vi "Init Hardware.vi"(8 "error in (no error)":errorcluster, 11 "Red Pitaya Digitizer in":refnum<class "Red Pitaya Digitizer.lvclass">) -> (0 "error out":errorcluster, 3 "Red Pitaya Digitizer out":refnum<class "Red Pitaya Digitizer.lvclass">)   [LabVIEW 2018, in "Red Pitaya Digitizer.lvclass"]
uses:
  Red Pitaya Digitizer.lvclass
  C:/github/NHMFL_Core/Libraries/Instruments/Pulse Driver/Pulse Driver.lvclass
  Red Pitaya Digitizer.lvclass/Red Pitaya Digitizer.ctl
  Instruments/Pulse Driver/Pulse Driver.lvclass/Pulse Driver.ctl
  RP Core/RP Instrument/RP Instrument.lvclass/RP Instrument.ctl
  RP Command.ctl
  Read Logic tag.vi
  Read RP Instrument.vi
  Instruments/Pulse Driver/Read Samples per channel.vi
  Instruments/Pulse Driver/Read Pretrigger samples.vi
  Read Tigger level.vi
  RP Core/RP Instrument/Write Decimation.vi
  RP Core/RP Instrument/Write Post-trigger samples.vi
  RP Core/RP Instrument/Write Samples per trigger increment .vi
  Write RP Instrument.vi
  Instruments/Pulse Driver/Write dt.vi
  Instruments/Pulse Driver/Write t0.vi
  Write Signal bits.vi
  Read Server address.vi
  RP Core/RP Instrument/RP Instrument.lvclass
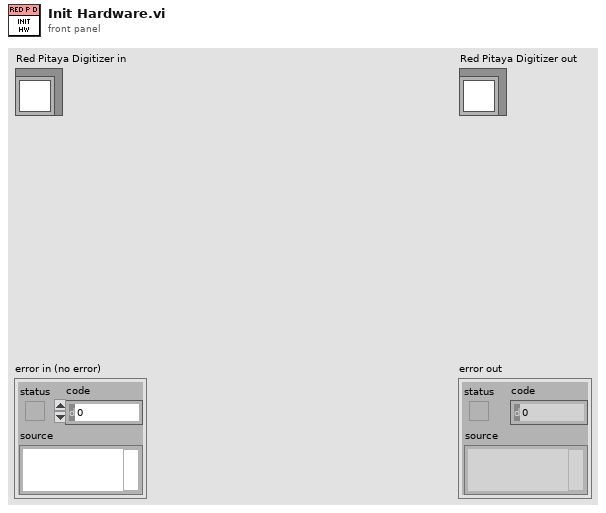
[diagram p1: front panel]
types:
  T1 = typedef "RP Command.ctl" = enum16{"Reset", "Read IDN", "Stop server", "Get status", "Get temperature", "Connect client", "Arm", "Software trigger", "Get whole buffer", "Get chunk", "System call", "Get config", "Set config", "Recieve data", "Recieve Calibartion", "Transmit data"}
  T2 = typedef "Pusle Driver Configuration.ctl" = cluster{"Pre-trigger duration":dbl, "Post-trigger duration":dbl, "Rate":dbl, "Ranges":dbl[], "Re-name channels":string[], "Active channels":string, "External clock":bool}
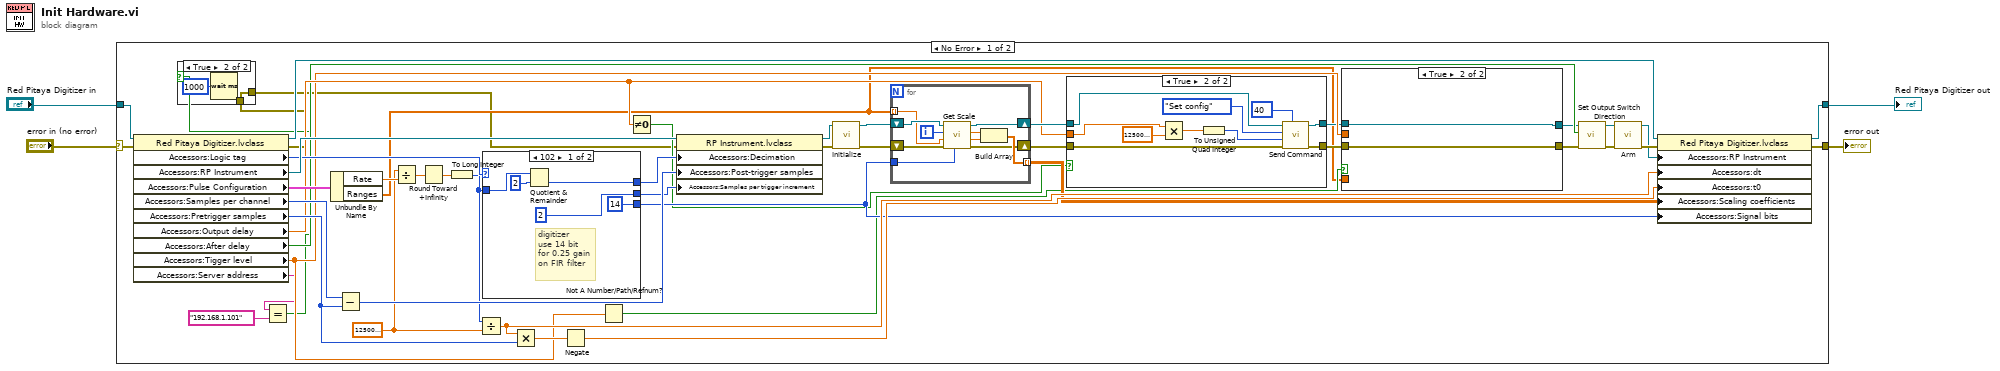
[diagram p0: block diagram]
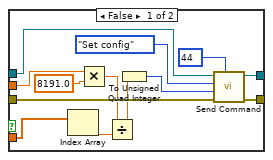
[diagram p3: hidden frame]
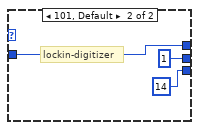
[diagram p5: hidden frame]
diagram:
  n1 = case shown="No Error" "error in (no error)" {
    selector: "error in (no error)" -> [w32 w101]
    tunnel: "Red Pitaya Digitizer in" -> [w52 w102]
    tunnel: [w40 w101] -> w2
    tunnel: [w39 w102] -> w1
    frame No Error {
      w38 = 125000000.0 ("y")
      n2 = property class="Red Pitaya Digitizer.lvclass"(reference=w52, error in=w32) -> (reference out=w42:refnum<class "Red Pitaya Digitizer.lvclass">, error out=w6:errorcluster, "Accessors:Logic tag"=w28:u16, "Accessors:RP Instrument"=w31:refnum<class "RP Instrument.lvclass">, "Accessors:Pulse Configuration"=w51:T2, "Accessors:Samples per channel"=w46:i32, "Accessors:Pretrigger samples"=w36:u32, "Accessors:Output delay"=w20:dbl, "Accessors:After delay"=w17:bool, "Accessors:Tigger level"=w12:dbl, "Accessors:Server address"=w9:string)
      n3 = Equal?(x=w9, y="192.168.1.101") -> (x = y?=w7:bool)
      n4 = case shown="True" w7 {
        tunnel: w6 -> [w53 w54]
        tunnel: [w53 w54] -> w5
        frame False {
        }
        frame True {
          n5 = Wait (ms)(milliseconds to wait=u32 1000) -> ()  [unwired: 1 out]
        }
      }
      n6 = Unbundle By Name(w51) -> ("Rate"=w50:dbl, "Ranges"=w10:dbl[])
      n7 = Subtract(x=w46, y=w36) -> (x-y=w45:u32)
      n8 = Divide(x=w38, y=w50) -> (x/y=w49:dbl)
      n9 = Round Toward +Infinity(x=w49) -> (ceil(x): smallest int >= x=w48:dbl)
      n10 = To Long Integer(number=w48) -> (32bit integer=w27:i32)
      n11 = Divide(x=w27, y=w38) -> (x/y=w37:dbl)
      n12 = case shown="102" w28 {
        tunnel: [14 ("Signal bits") 14 ("Signal bits")] -> w29
        tunnel: [2 ("Samples per trigger increment") 1 ("Samples per trigger increment")] -> w30
        tunnel: w27 -> [w85 w88]
        tunnel: [w83 w88] -> w26
        frame 102 {
          # "digitizer\nuse 14 bit \nfor 0.25 gain\non FIR filter"
          n13 = Quotient & Remainder(x=w85, y=2) -> (floor(x/y)=w83:i32)  [unwired: 1 out]
        }
        frame 101, Default {
          # "lockin-digitizer"
        }
      }
      n14 = Multiply(x=w37, y=w36) -> (x*y=w35:dbl)
      n15 = Negate(x=w35) -> (-x=w34:dbl)
      n16 = Not A Number/Path/Refnum?(number/path/refnum=w12) -> (NaN/Path/Refnum?=w13:bool)
      n17 = Not Equal To 0?(x=w20) -> (x != 0?=w23:bool)
      n18 = property class="RP Instrument.lvclass"(reference=w31, error in=w5, "Accessors:Decimation"=w26, "Accessors:Post-trigger samples"=w45, "Accessors:Samples per trigger increment "=w30) -> (reference out=w47:refnum<class "RP Instrument.lvclass">, error out=w44:errorcluster)
      n19 = call-dynamic "Initialize.vi"("error in (no error)"=w44, "RP Instrument in"=w47) -> ("error out"=w24:errorcluster, "RP Instrument out"=w25:refnum<class "RP Instrument.lvclass">)  [unwired: 8 in]
      n20 = for {
        tunnel: w10 -> [w92] mode=indexing
        tunnel: [w100] -> w33 mode=indexing
        tunnel: w29 -> [w91]
        shift-right: [w98] -> w21
        shift-left: w25 -> [w99]
        shift-right: [w96] -> w22
        shift-left: w24 -> [w97]
        i -> [w93]
        n21 = call-dynamic "Get Scale.vi"("Signal bits"=w91, "error in (no error)"=w97, "Range"=w92, "Channel"=w93, "RP Instrument in"=w99) -> ("error out"=w96:errorcluster, "slope"=w94:dbl, "y intersept"=w95:dbl, "RP Instrument out"=w98:refnum<class "RP Instrument.lvclass">)  [unwired: 2 in, 1 out]
        n22 = Build Array(w95, w94) -> (w100:dbl[])
      }
      n23 = case shown="True" w23 {
        tunnel: w22 -> [w71 w77]
        tunnel: w21 -> [w72 w76]
        tunnel: w20 -> [_ w75]
        tunnel: [w71 w74] -> w16
        tunnel: [w72 w73] -> w11
        frame False {
        }
        frame True {
          n24 = Multiply(x=w75, y=125000000.0) -> (x*y=w81:dbl)
          n25 = To Unsigned Quad Integer(1:w81) -> (0:w82:u64)
          n26 = call-dynamic "Send Command.vi"("Config offset"=u64 40, "error in (no error)"=w77, "Command payload"=w82, "Command number"=RP_Command."Set config", "RP Instrument in"=w76) -> ("error out"=w74:errorcluster, "RP Instrument out"=w73:refnum<class "RP Instrument.lvclass">)  [unwired: 5 in]
        }
      }
      n27 = case shown="True" w13 {
        tunnel: w16 -> [w64 w69]
        tunnel: w11 -> [w60 w70]
        tunnel: w12 -> [w63 _]
        tunnel: [w62 w69] -> w15
        tunnel: [w61 w70] -> w14
        tunnel: w10 -> [w59 _]
        frame False {
          n28 = Index Array(array=w59) -> (element=w56:dbl)  [unwired: 1 in]
          n29 = Multiply(x=w63, y=8191.0) -> (x*y=w57:dbl)
          n30 = Divide(x=w57, y=w56) -> (x/y=w58:dbl)
          n31 = To Unsigned Quad Integer(1:w58) -> (0:w68:u64)
          n32 = call-dynamic "Send Command.vi"("Config offset"=u64 44, "error in (no error)"=w64, "Command payload"=w68, "Command number"=RP_Command."Set config", "RP Instrument in"=w60) -> ("error out"=w62:errorcluster, "RP Instrument out"=w61:refnum<class "RP Instrument.lvclass">)  [unwired: 5 in]
        }
        frame True {
        }
      }
      n33 = call-dynamic "Set Output Switch Direction.vi"("error in (no error)"=w15, "After delay"=w17, "RP Instrument in"=w14) -> ("error out"=w19:errorcluster, "RP Instrument out"=w18:refnum<class "RP Instrument.lvclass">)  [unwired: 7 in]
      n34 = call-dynamic "Arm.vi"("error in (no error)"=w19, "RP Instrument in"=w18) -> ("error out"=w43:errorcluster, "RP Instrument out"=w41:refnum<class "RP Instrument.lvclass">)  [unwired: 8 in]
      n35 = property class="Red Pitaya Digitizer.lvclass"(reference=w42, error in=w43, "Accessors:RP Instrument"=w41, "Accessors:dt"=w37, "Accessors:t0"=w34, "Accessors:Scaling coefficients"=w33, "Accessors:Signal bits"=w29) -> (reference out=w39:refnum<class "Red Pitaya Digitizer.lvclass">, error out=w40:errorcluster)
    }
    frame Error {
    }
  }
  "error out" <- w2
  "Red Pitaya Digitizer out" <- w1
